vi "MW_Display_Py_Set_Configuration.vi"(0 "session in":refnum<k35>, 5 "module path":path=path "D:/dev/Guy_Storage/Work/Cancun/MW_Display_Test/Magewell Capture/Capture_LV.py", 11 "error in":errorcluster, 12 "Configuration":T2) -> (4 "session out":refnum<k35>, 6 "module path out":path, 14 "Done":T1, 15 "error out":errorcluster)   [LabVIEW 2023]
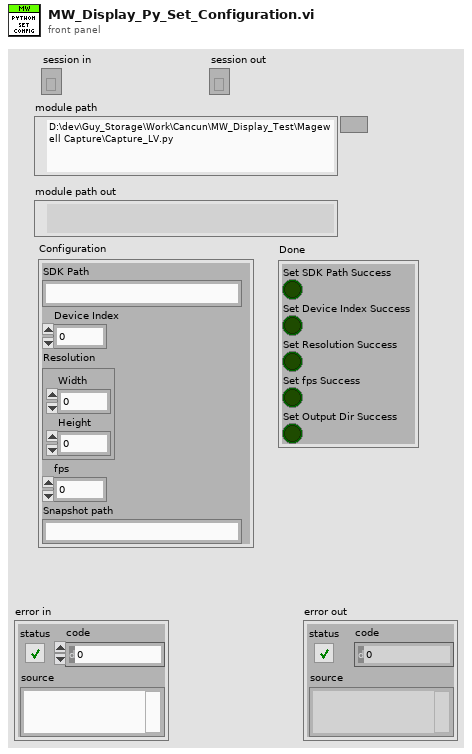
[diagram p1: front panel]
types:
  T1 = cluster{"Set SDK Path Success":bool, "Set Device Index Success":bool, "Set Resolution Success":bool, "Set fps Success":bool, "Set Output Dir Success":bool}
  T2 = cluster{"SDK Path":string, "Device Index":i32, "Resolution":cluster{"Width":i32, "Height":i32}, "fps":i32, "Snapshot path":string}
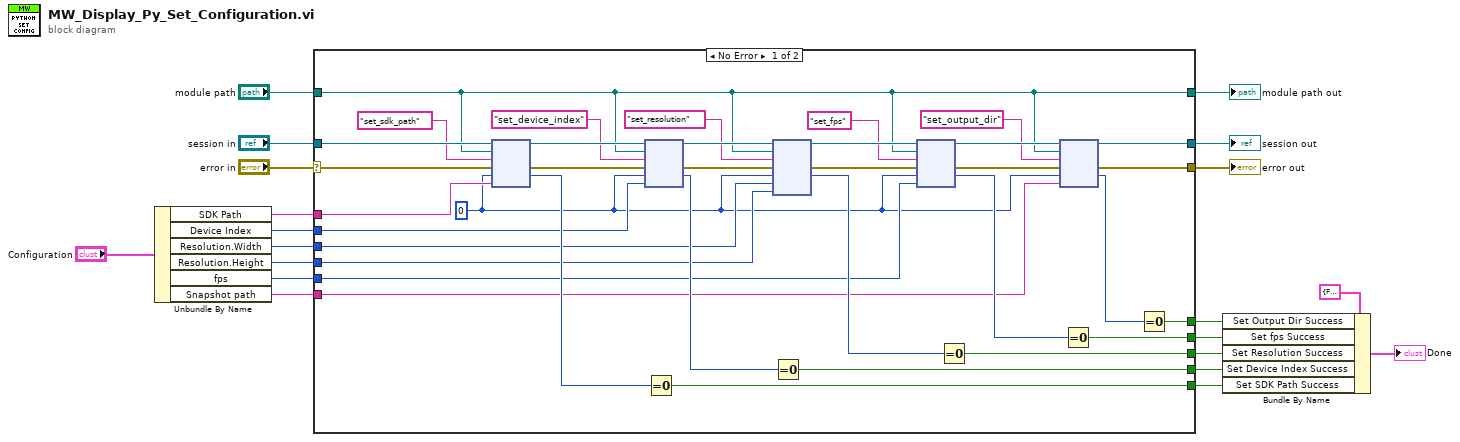
[diagram p0: block diagram]
diagram:
  n1 = Unbundle By Name("Configuration") -> ("SDK Path"=w13:string, "Device Index"=w12:i32, "Resolution.Width"=w11:i32, "Resolution.Height"=w10:i32, "fps"=w9:i32, "Snapshot path"=w8:string)
  n2 = case shown="No Error" "error in" {
    selector: "error in" -> [w54 w57]
    tunnel: "module path" -> [w28 w56]
    tunnel: "session in" -> [w55 w58]
    tunnel: [w22 w57] -> w16
    tunnel: [w21 w58] -> w18
    tunnel: [w28 w56] -> w15
    tunnel: w13 -> [w52 _]
    tunnel: [w50 _] -> w2
    tunnel: w12 -> [w46 _]
    tunnel: [w44 _] -> w3
    tunnel: w11 -> [w40 _]
    tunnel: w10 -> [w39 _]
    tunnel: [w37 _] -> w4
    tunnel: w9 -> [w33 _]
    tunnel: [w31 _] -> w5
    tunnel: w8 -> [w26 _]
    tunnel: [w23 _] -> w6
    frame No Error {
      w25 = 0
      n3 = node(w55, w28, "set_sdk_path" ("function name"), w54, w25, w52) -> (w48:refnum<k35>, w49:errorcluster, w51:i32)  [unwired: 1 in, 2 out]
      n4 = node(w48, w28, "set_device_index" ("function name"), w49, w25, w46) -> (w42:refnum<k35>, w43:errorcluster, w45:i32)  [unwired: 1 in, 2 out]
      n5 = Equal To 0?(x=w51) -> (x = 0?=w50:bool)
      n6 = node(w42, w28, "set_resolution" ("function name"), w43, w25, w40, w39) -> (w36:refnum<k35>, w35:errorcluster, w38:i32)  [unwired: 2 in, 2 out]
      n7 = Equal To 0?(x=w45) -> (x = 0?=w44:bool)
      n8 = node(w36, w28, "set_fps" ("function name"), w35, w25, w33) -> (w30:refnum<k35>, w29:errorcluster, w32:i32)  [unwired: 1 in, 2 out]
      n9 = Equal To 0?(x=w38) -> (x = 0?=w37:bool)
      n10 = node(w30, w28, "set_output_dir" ("function name"), w29, w25, w26) -> (w21:refnum<k35>, w22:errorcluster, w24:i32)  [unwired: 1 in, 2 out]
      n11 = Equal To 0?(x=w32) -> (x = 0?=w31:bool)
      n12 = Equal To 0?(x=w24) -> (x = 0?=w23:bool)
    }
    frame Error {
    }
  }
  "session out" <- w18
  "error out" <- w16
  "module path out" <- w15
  n13 = Bundle By Name(cluster=T1 {"Set SDK Path Success"=FALSE, "Set Device Index Success"=FALSE, "Set Resolution Success"=FALSE, "Set fps Success"=FALSE, "Set Output Dir Success"=FALSE} ("Done"), "Set Output Dir Success"=w6, "Set fps Success"=w5, "Set Resolution Success"=w4, "Set Device Index Success"=w3, "Set SDK Path Success"=w2) -> (→"Done":T1)
